vi "range_wrap.vi"(0 "Array":dbl[][](array[numeric]), 2 "upper limit":dbl=1.0 format="%#_13g") -> (8 "Array output":dbl[][](array[numeric]))   [LabVIEW 2020]
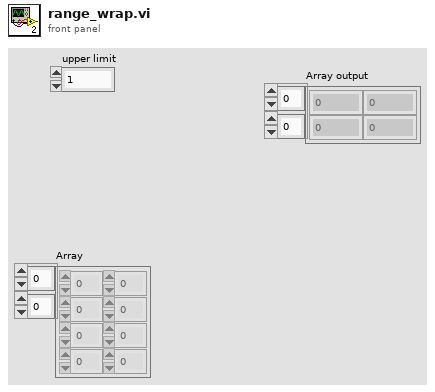
[diagram p1: front panel]
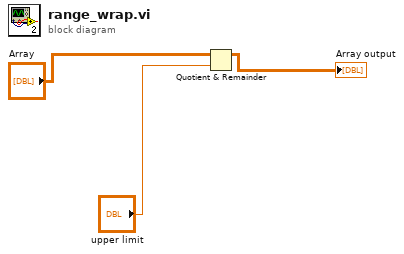
[diagram p0: block diagram]
diagram:
  n1 = Quotient & Remainder(x="Array", y="upper limit") -> (x-y*floor(x/y)=→"Array output":dbl[][])  [unwired: 1 out]
